vi "RemoveBackgrund2D.vi"(7 "Expected FWHM (xy)":dbl=2.2, 11 "sum xy":i32[][](graph)) -> (3 "sum xy 2":i32[][](graph))   [LabVIEW 2011]
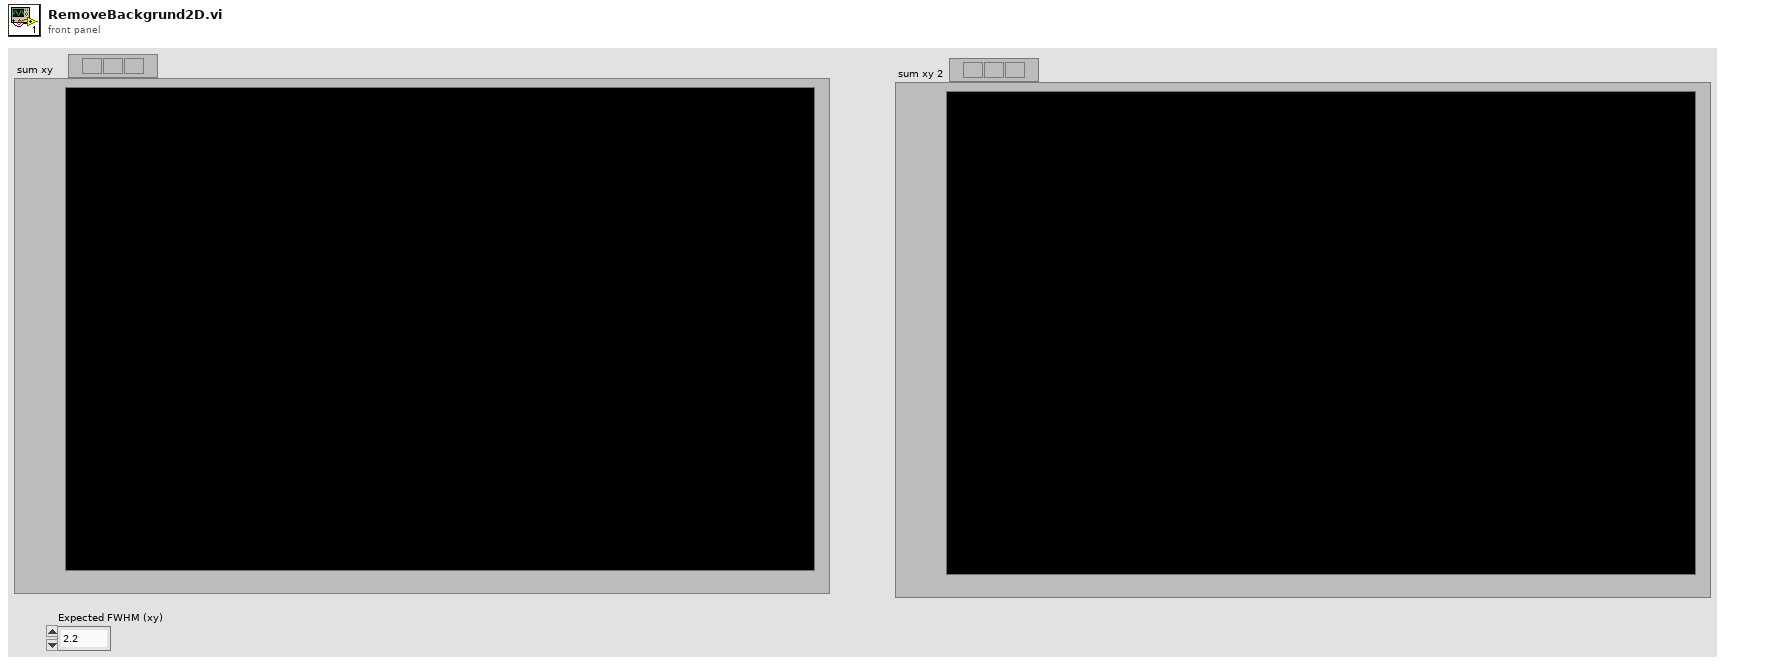
[diagram p1: front panel]
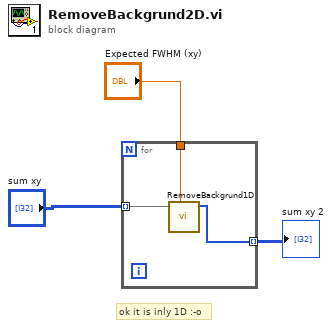
[diagram p0: block diagram]
diagram:
  # "ok it is inly 1D :-o"
  n1 = for {
    tunnel: "sum xy" -> [w6] mode=indexing
    tunnel: [w5] -> w2 mode=indexing
    tunnel: "Expected FWHM (xy)" -> [w4]
    n2 = call "RemoveBackgrund1D.vi"("Expected FWHM (xy)"=w4, "Waveform Graph"=w6) -> ("Waveform Graph 3"=w5:i32[])  [unwired: 9 in]
  }
  "sum xy 2" <- w2
